vi "get Class Data.vi"(8 "Error In":errorcluster, 10 "Selected Instance":string, 11 "Instance Data Array":T1[](array[typedef])) -> (0 "Error Out":errorcluster)   [LabVIEW 2023, in "Arithemetic Operation.lvclass"]
doc: "This method gets the data of the instance searched by the user."
uses:
  Arithemetic Operation.lvclass
  Typedef/Class Data.ctl
  Typedef/User Event Operations.ctl
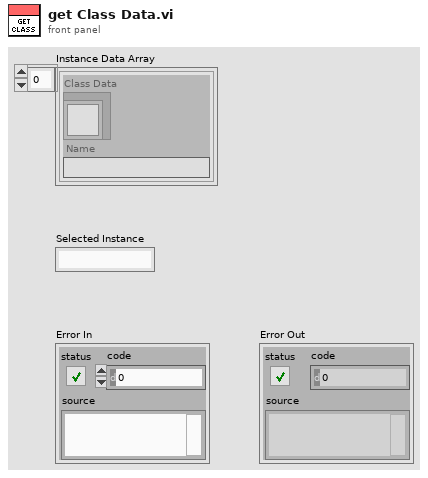
[diagram p1: front panel]
types:
  T1 = typedef "Class Data.ctl" = cluster{"Class Data":refnum<class "Arithemetic Operation.lvclass">, "Name":string}
  T2 = typedef "User Event Operations.ctl" = enum16{"Obtain", "Generate", "Release"}
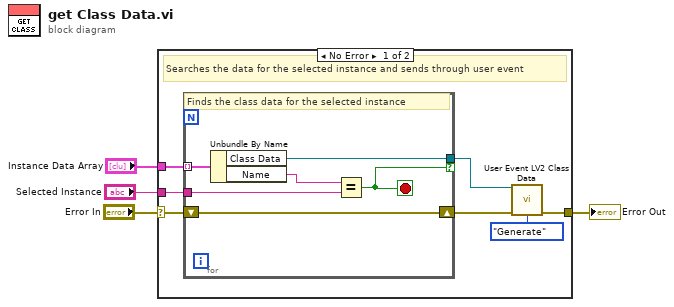
[diagram p0: block diagram]
diagram:
  n1 = case shown="No Error" "Error In" {
    selector: "Error In" -> [w7 w18]
    tunnel: [w8 w18] -> w3
    tunnel: "Instance Data Array" -> [w6 _]
    tunnel: "Selected Instance" -> [w5 _]
    frame No Error {
      # "Searches the data for the selected instance and sends through user event"
      n2 = for {
        tunnel: w6 -> [w17] mode=indexing
        tunnel: [w15] -> w9 if=w13
        tunnel: w5 -> [w12]
        shift-right: [w14] -> w11
        shift-left: w7 -> [w14]
        stop <- w13 stop-if-true
        # "Finds the class data for the selected instance"
        n3 = Unbundle By Name(w17) -> ("Class Data"=w15:refnum<class "Arithemetic Operation.lvclass">, "Name"=w16:string)
        n4 = Equal?(x=w16, y=w12) -> (x = y?=w13:bool)
      }
      n5 = call "User Event LV2 Class Data.vi"("Class Data"=w9, "Error In"=w11, "Operation"=User_Event_Operations."Generate") -> ("Error Out"=w8:errorcluster)  [unwired: 11 in, 1 out]
    }
    frame Error {
    }
  }
  "Error Out" <- w3
